vi "Test Write Read Library Icon Data.vi"(11 "Test Case In":refnum<class "Library Icon Data.lvclass">) -> (0 "error out":errorcluster, 3 "Test Case Out":refnum<class "Library Icon Data.lvclass">)   [LabVIEW 2020, in "Library Icon Data.lvclass"]
uses:
  Library Icon Data.lvclass
  vi.lib/LabVIEW Icon API/lv_icon/Controls/LabVIEW Icon Stored Information.ctl
  vi.lib/LabVIEW Icon API/lv_icon/Classes/Layer/Layer.lvclass
  vi.lib/LabVIEW Icon API/lv_icon/Controls/BodyText.ctl
  vi.lib/LabVIEW Icon API/lv_icon/Controls/Font.ctl
  vi.lib/LabVIEW Icon API/lv_icon/Controls/Alignment.ctl
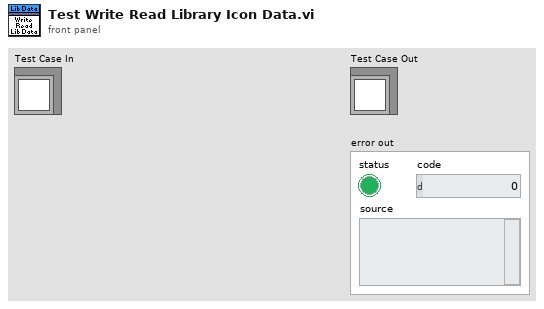
[diagram p1: front panel]
types:
  T1 = typedef "LabVIEW Icon Stored Information.ctl" = cluster{"Text Visible?":bool, "Text Opacity":u8, "Templ Visible?":bool, "Templ Opacity":u8, "Relative Path from 1 to 2":path, "Image":picture, "All User Layers":refnum<class "Layer.lvclass">[], "Body Text":T2}
  T2 = typedef "BodyText.ctl" = cluster{"Line 1 text":string, "Line 2 text":string, "Line 3 text":string, "Line 4 text":string, "Line 1 color":u32, "Line 2 color":u32, "Line 3 color":u32, "Line 4 color":u32, "Body Text Spec":cluster{"Font":T3, "Alignment":T4, "Size":u8}, "Center text vertically":bool, "Capitalize Text":bool}
  T3 = typedef "Font.ctl" = string
  T4 = typedef "Alignment.ctl" = u16
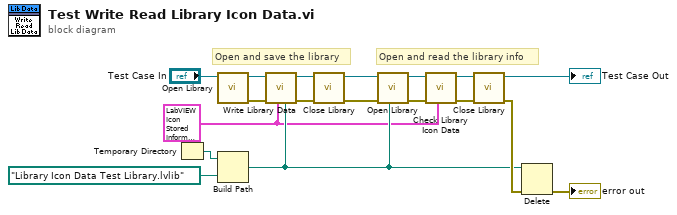
[diagram p0: block diagram]
diagram:
  w1 = T1 {"Text Visible?"=TRUE, "Text Opacity"=100, "Templ Visible?"=TRUE, "Templ Opacity"=100, "Relative Path from 1 to 2"=path "Library/3rd party/Library Header.png", "Image"=bytes[3230], "All User Layers"=[refnum], "Body Text"={"Line 1 text"="LVLib", "Line 2 text"="", "Line 3 text"="", "Line 4 text"="", "Line 1 color"=16711680, "Line 2 color"=0, "Line 3 color"=0, "Line 4 color"=0, "Body Text Spec"={"Font"="Small Fonts", "Alignment"=1, "Size"=8}, "Center text vertically"=TRUE, "Capitalize Text"=FALSE}} ("Icon data")
  # "Open and read the library info"
  # "Open and save the library"
  n1 = Temporary Directory() -> (w11:path)
  n2 = call "Open Library.vi"("Library Icon Data in"="Test Case In") -> ("error out"=w18:errorcluster, "Library Icon Data out"=w8:refnum<class "Library Icon Data.lvclass">)  [unwired: 9 in]
  n3 = Build Path(base path=w11, name or relative path=path "Library Icon Data Test Library.lvlib") -> (appended path=w2:path)
  n4 = call "Write Library Data.vi"("Library Path"=w2, "Icon data"=w1, "error in"=w18, "Library Icon Data in"=w8) -> ("error out"=w17:errorcluster, "Library Icon Data out"=w7:refnum<class "Library Icon Data.lvclass">)  [unwired: 6 in]
  n5 = call "Close Library.vi"("error in"=w17, "Library Icon Data in"=w7) -> ("error out"=w16:errorcluster, "Library Icon Data out"=w6:refnum<class "Library Icon Data.lvclass">)  [unwired: 8 in]
  n6 = call "Open Library.vi"("Library Path"=w2, "error in"=w16, "Library Icon Data in"=w6) -> ("error out"=w15:errorcluster, "Library Icon Data out"=w5:refnum<class "Library Icon Data.lvclass">)  [unwired: 7 in]
  n7 = call "Check Library Icon Data.vi"("Expected Icon data"=w1, "error in"=w15, "Library Icon Data in"=w5) -> ("error out"=w14:errorcluster, "Library Icon Data out"=w4:refnum<class "Library Icon Data.lvclass">)  [unwired: 7 in]
  n8 = call "Close Library.vi"("error in"=w14, "Library Icon Data in"=w4) -> ("error out"=w13:errorcluster, "Library Icon Data out"=→"Test Case Out":refnum<class "Library Icon Data.lvclass">)  [unwired: 8 in]
  n9 = Delete(path (use dialog)=w2, error in=w13) -> (error out=→"error out":errorcluster)  [unwired: 3 in, 2 out]
